vi "Excel Sheet Read.vi"(8 "error in (no error)":errorcluster, 9 "Name(\"\")":string, 10 "Index(1)":i32=1, 11 "Excel Path":path=path "D:/SVN_DKY/TestFile/116 2MW/@IO点表/116点表 - 20160315.xlsx") -> (0 "error out":errorcluster, 3 "Data":string[][](array[string]))   [LabVIEW 2013]
uses:
  <vilib>/K2Labs/HiLab API/Custom Device API/Custom Device API Library.lvlib
panel:
  in  "Excel._Application":refnum<k7>
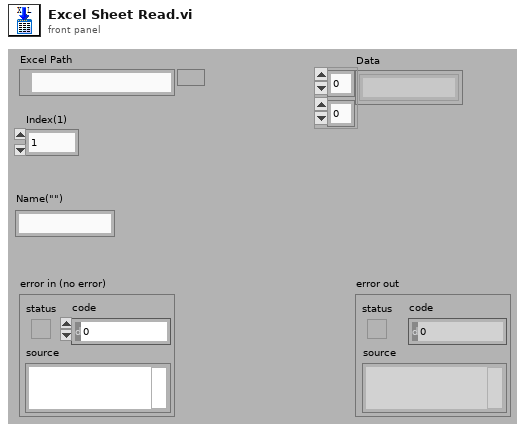
[diagram p1: front panel]
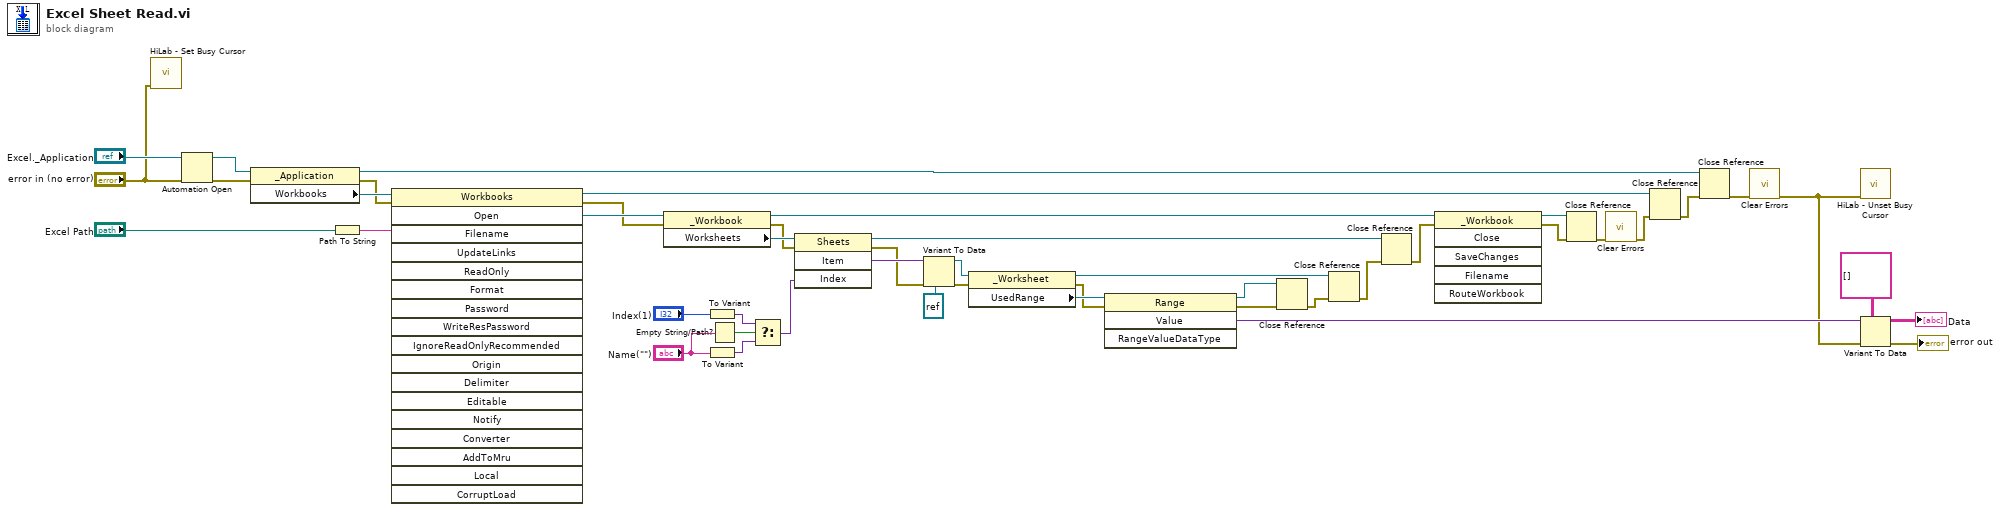
[diagram p0: block diagram]
diagram:
  n1 = call <vilib>:"HiLab - Set Busy Cursor.vi"("error in (no error)"="error in (no error)") -> ()  [unwired: 10 in, 1 out]
  n2 = Automation Open(error in (no error)="error in (no error)", Automation Refnum="Excel._Application") -> (Automation Refnum=w40:refnum<k7>, error out=w31:errorcluster)  [unwired: 2 in]
  n3 = property class="_Application"(reference=w40, error in=w31) -> (reference out=w8:refnum<k7>, error out=w30:errorcluster, "Workbooks"=w46:refnum<k7>)
  n4 = Path To String(path="Excel Path") -> (string=w45:string)
  n5 = invoke class="Workbooks" method="Open"(reference=w46, error in=w30, "Filename"=w45) -> (reference out=w23:refnum<k7>, error out=w29:errorcluster, "Open"=w43:refnum<k7>)  [unwired: 15 in, 15 out]
  n6 = property class="_Workbook"(reference=w43, error in=w29) -> (reference out=w22:refnum<k7>, error out=w28:errorcluster, "Worksheets"=w39:refnum<k7>)
  n7 = To Variant(anything="Index(1)") -> (Variant=w13:variant)
  n8 = To Variant(anything="Name(\"\")") -> (Variant=w11:variant)
  n9 = Empty String/Path?(string/path="Name(\"\")") -> (empty?=w14:bool)
  n10 = Select(t=w13, s=w14, f=w11) -> (s? t:f=w10:variant)
  n11 = invoke class="Sheets" method="Item"(reference=w39, error in=w28, "Index"=w10) -> (reference out=w21:refnum<k7>, error out=w27:errorcluster, "Item"=w42:variant)  [unwired: 1 in, 1 out]
  n12 = Variant To Data(error in=w27, type=refnum<k7> refnum ("Excel._Worksheet"), Variant=w42) -> (data=w37:refnum<k7>, error out=w26:errorcluster)
  n13 = property class="_Worksheet"(reference=w37, error in=w26) -> (reference out=w20:refnum<k7>, error out=w25:errorcluster, "UsedRange"=w36:refnum<k7>)
  n14 = invoke class="Range" method="Value"(reference=w36, error in=w25) -> (reference out=w19:refnum<k7>, error out=w16:errorcluster, "Value"=w35:variant)  [unwired: 2 in, 1 out]
  n15 = Close Reference(reference=w19, error in (no error)=w16) -> (error out=w17:errorcluster)
  n16 = Close Reference(reference=w20, error in (no error)=w17) -> (error out=w18:errorcluster)
  n17 = Close Reference(reference=w21, error in (no error)=w18) -> (error out=w5:errorcluster)
  n18 = invoke on="调用节点" class="_Workbook" method="Close"(reference=w22, error in=w5) -> (reference out=w6:refnum<k7>, error out=w4:errorcluster)  [unwired: 4 in, 4 out]
  n19 = Close Reference(reference=w6, error in (no error)=w4) -> (error out=w15:errorcluster)
  n20 = call <vilib>:"Clear Errors.vi"("error in (no error)"=w15) -> ("error out"=w3:errorcluster)  [unwired: 6 in]
  n21 = Close Reference(reference=w23, error in (no error)=w3) -> (error out=w7:errorcluster)
  n22 = Close Reference(reference=w8, error in (no error)=w7) -> (error out=w24:errorcluster)
  n23 = call <vilib>:"Clear Errors.vi"("error in (no error)"=w24) -> ("error out"=w1:errorcluster)  [unwired: 6 in]
  n24 = call <vilib>:"HiLab - Unset Busy Cursor.vi"("error in (no error)"=w1) -> ()  [unwired: 10 in, 1 out]
  n25 = Variant To Data(error in=w1, type=string[][] [], Variant=w35) -> (data=→"Data":string[][], error out=→"error out":errorcluster)
